vi "UHR-Fleezers Control (host) - 10.6.vi"() -> ()   [LabVIEW 2011] (continued)
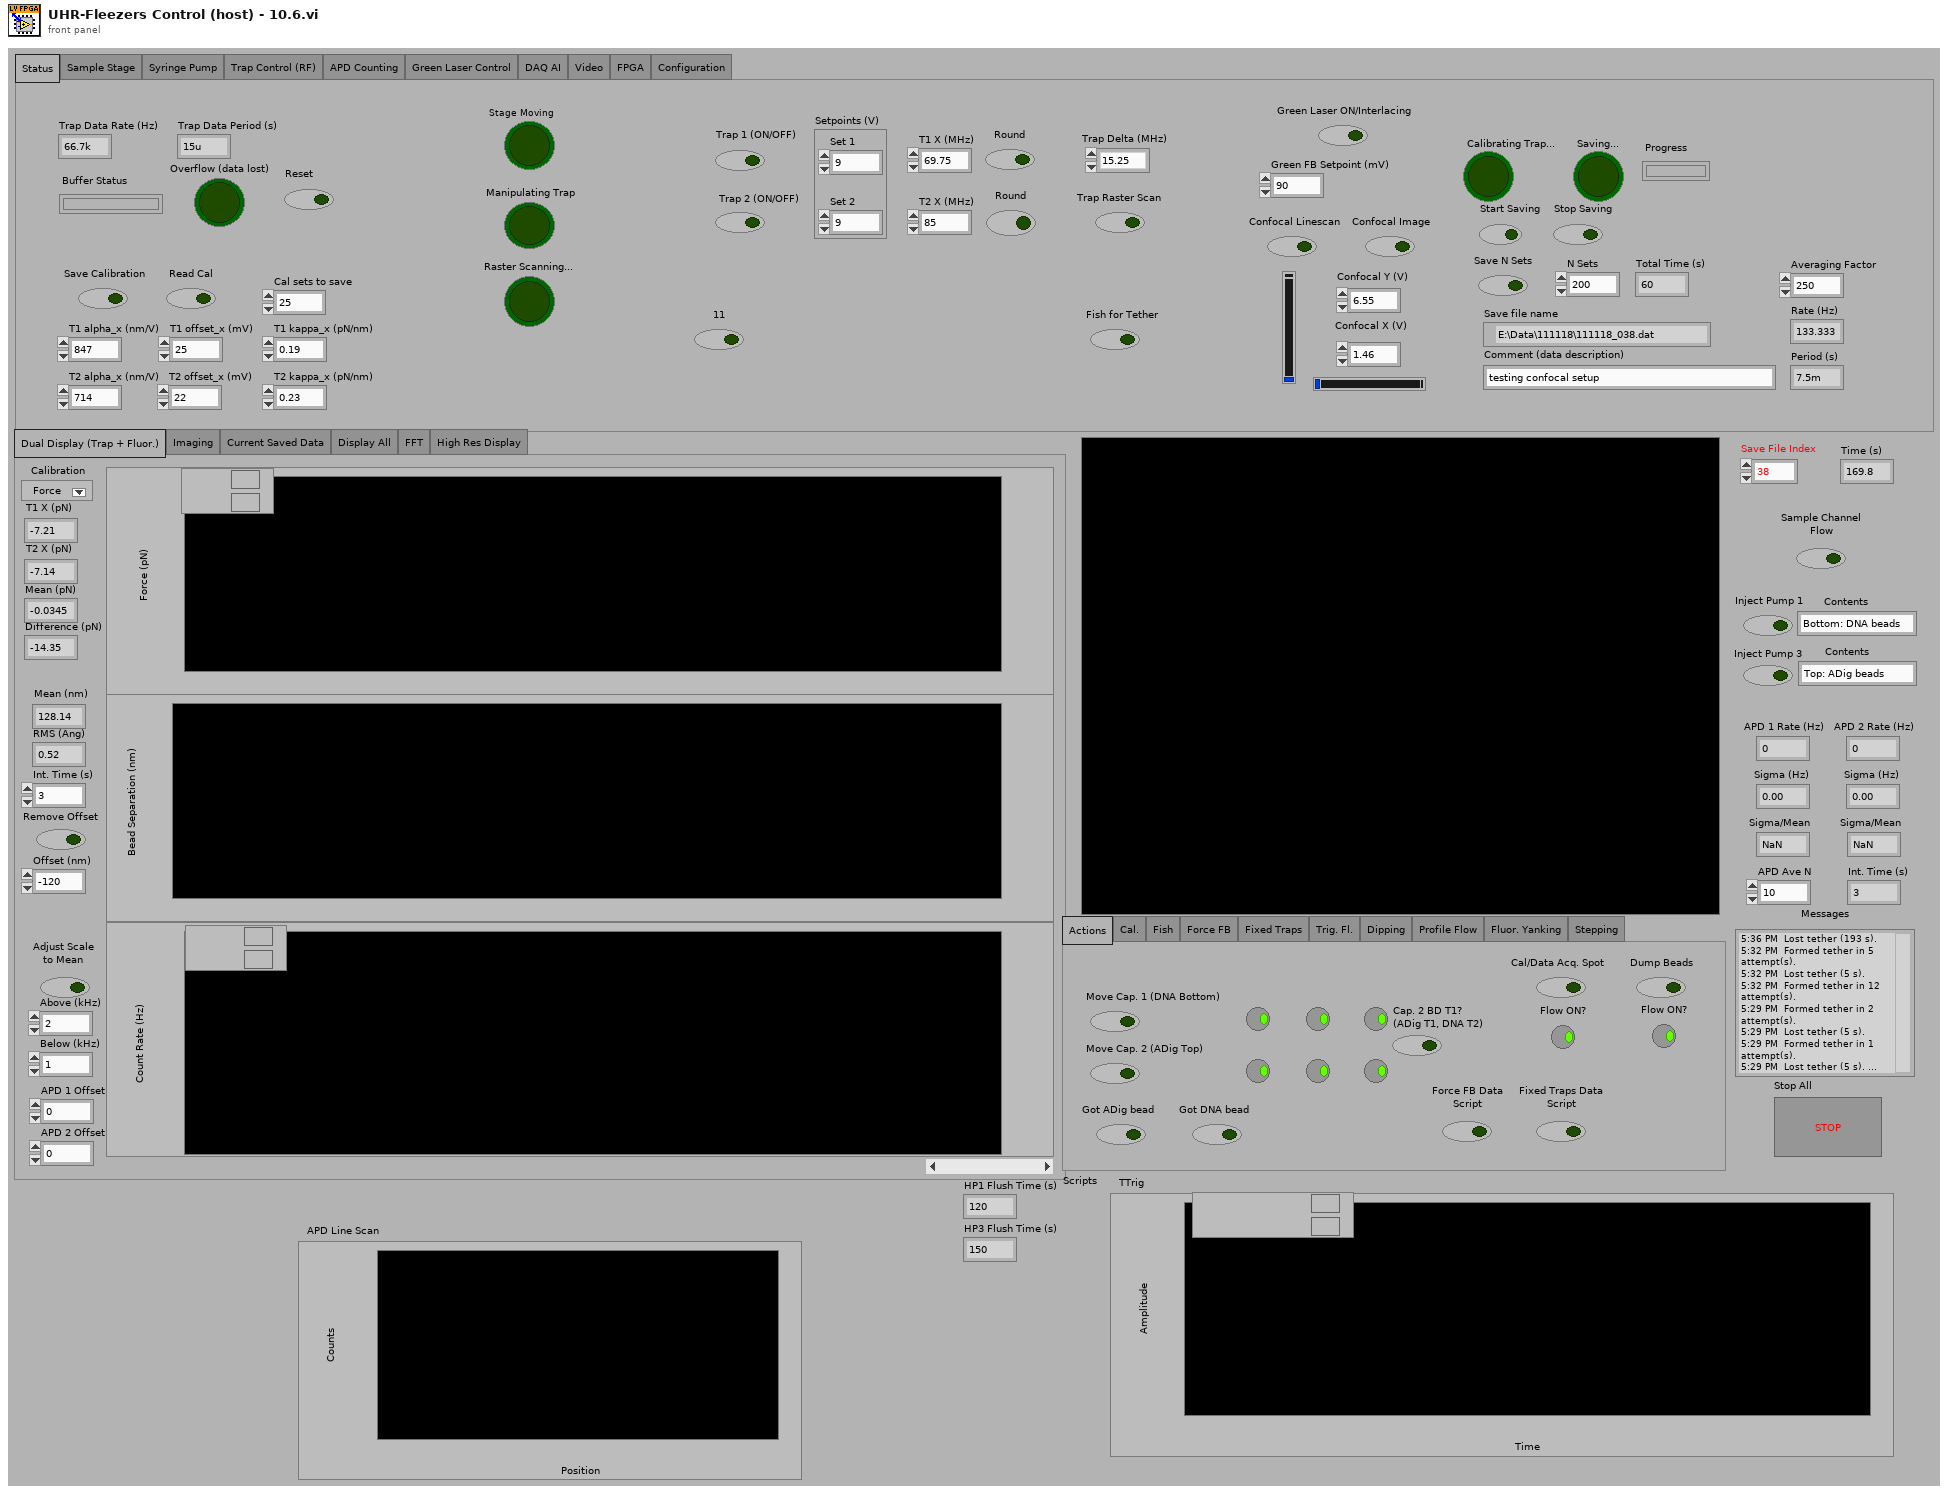
[diagram p1: front panel]
types:
  T1 = enum32{"Actions", "Cal.", "Fish", "Force FB", "Fixed Traps", "Trig. Fl.", "Dipping", "Profile Flow", "Fluor. Yanking", "Stepping"}
  T2 = typedef "IMAQ Image.ctl" = refnum<image>
  T3 = enum32{"Dual Display (Trap + Fluor.)", "Imaging", "Current Saved Data", "Display All", "FFT", "High Res Display"}
  T4 = enum32{"Status", "Sample Stage", "Syringe Pump", "Trap Control (RF)", "APD Counting", "Green Laser Control", "DAQ AI", "Video", "FPGA", "Configuration"}
  T5 = cluster{"Pump 1":cluster{"Diameter (mm)":dbl, "Units":dbl, "Volume":dbl, "Rate":dbl}, "Pump 2":cluster{"Diameter (mm)":dbl, "Units":dbl, "Volume":dbl, "Rate":dbl}, "Pump 3":cluster{"Diameter (mm)":dbl, "Units":dbl, "Volume":dbl, "Rate":dbl}}
  T6 = enum32{"IR Laser Interlacing (Direct RF Board Control Method)", "AOD Raster Scan", "Feedback on Trap Intensity", "Feedback on Trap Position"}
  T7 = typedef "LVPoint32TypeDef.ctl" = cluster{"Horizontal":i32, "Vertical":i32}
  T8 = cluster{"Scan Range AOD (nm) 2":dbl, "Step Size AOD (nm) 2":dbl, "Scan Speed AOD (nm/s) 2":dbl, "Number of scans (AOD) 2":u16, "Label":string}[]
  T9 = cluster{"Set 1":cluster{"proportional gain (Kc)":i16, "integral gain (Kc*Ts/Ti)":i16, "derivative gain (Kc*Td/Ts)":i16}, "Set 2":cluster{"proportional gain (Kc)":i16, "integral gain (Kc*Ts/Ti)":i16, "derivative gain (Kc*Td/Ts)":i16}}
  T10 = cluster{"Trap 1":fxp<+/-,16,1>, "Trap 2":fxp<+/-,16,1>}
  T11 = cluster{"proportional gain (Kc)":fxp<+/-,16,8>, "integral gain (Kc*Ts/Ti)":fxp<+/-,16,8>, "derivative gain (Kc*Td/Ts)":fxp<+/-,16,8>}
  T12 = cluster{"output high":fxp<+/-,16,1>, "output low":fxp<+/-,16,1>}
  T13 = cluster{"Set 1":fxp<+/-,16,1>, "Set 2":fxp<+/-,16,1>}
  T14 = cluster{"proportional gain (Kc)":i16, "integral gain (Kc*Ts/Ti)":i16, "derivative gain (Kc*Td/Ts)":i16}
  T15 = cluster{"Set 1":bool, "Set 2":bool, "Set 3":bool}
  T16 = typedef "LVMinMaxIncTypeDef.ctl" = cluster{"Minimum":dbl, "Maximum":dbl, "Increment":dbl}
  T17 = typedef "Image Type" = u32
  T18 = typedef "nirio_resource_hc.ctl" = tag
  T19 = typedef "openfpgaref.8.6.ctl" = refnum<k20>
  T20 = cluster{"New Image":T2, "New Image":T2, "New Image":T2, "New Image":T2}
  T21 = typedef "XDNodeRunTimeDep.lvlib/timing_clust.ctl" = cluster{"Expected End [f-1]":u64, "Actual End [f-1]":u64, "Finished Late? [f-1]":bool, "Expected End [i-1]":u64, "Actual End [i-1]":u64, "Finished Late? [i-1]":bool, "Expected Start [i]":u64, "Actual Start [i]":u64, "Expected Start [f]":u64, "Actual Start [f]":u64, "Source Name":string, "Structure Name":string, "Period":i64, "Deadline":i64, "Offset":i64, "Start":i64, "Priority":i32, "Timeout":i32, "Mode":T22, "Wakeup Reason":T23, "Error":errorcluster, "Source Type":string, "Secondary Source Type":string, "Global End Time":u64, "Global Start Time":u64, "Frame Duration":u64, "Iteration Duration":u64, "Assigned CPU":i32, "I/O Scan Engine Mode":u32}
  T22 = typedef "XDNodeRunTimeDep.lvlib/nitl_modes.ctl" = enum32{"No Change", "Process missed periods, maintain original phase", "Discard missed periods, maintain original phase", "Process missed periods, ignore original phase", "Discard missed periods, ignore original phase"}
  T23 = typedef "XDNodeRunTimeDep.lvlib/wakeup.ctl" = enum32{"Normal", "Aborted", "Asynchronous wakeup", "Timing source error", "Timed loop error", "Timeout"}
  T24 = enum16{"big-endian, network order", "native, host order", "little-endian"}
  T25 = enum16{"open", "replace", "create", "open or create", "replace or create", "replace or create with confirmation"}
  T26 = cluster{"Scan Range AOD (nm) 2":dbl, "Step Size AOD (nm) 2":dbl, "Scan Speed AOD (nm/s) 2":dbl, "Number of scans (AOD) 2":u16, "Label":string}
  T27 = cluster{"[0]":dbl, "[1]":dbl, "[2]":dbl, "[3]":dbl, "[4]":dbl, "[5]":dbl}
  T28 = cluster{"Diameter (mm)":dbl, "Units":dbl, "Volume":dbl, "Rate":dbl}
  T29 = cluster{"Left":i32, "Top":i32, "Width":u32, "Height":u32}
  T30 = cluster{cluster{"Left":i32, "Top":i32, "Width":u32, "Height":u32}}[]
  T31 = enum32{"setting", "request", "request control", "info", "statistics", "system settings", "I/O sub system", "HRT control", "camera descriptions", "device specific data", "event sub system settings", "event sub system results", "image memory manager"}
  T32 = typedef "AviRefnum.ctl" = refnum<k1>
  T33 = typedef "imagedata.ctl" = cluster{"image type":i32, "image depth":i32, "image":u8[], "mask":u8[], "colors":u32[], "Rectangle":cluster{"left":i16, "top":i16, "right":i16, "bottom":i16}}
  T34 = enum32{"Normal Display", "Dual Display (APD)", "FFT", "High Res Display"}
  T35 = cluster{"Origin Pixel":cluster{"X":sgl, "Y":sgl}, "Angle Relative to Horizontal (deg)":sgl, "Axis Reference":u32}
  T36 = typedef "Simple Grid Descriptor" = cluster{"X Step":sgl, "Y Step":sgl, "Unit":T37}
  T37 = typedef "Image Unit" = enum32{"Undefined", "Angström", "Micrometer", "Millimeter", "Centimeter", "Meter", "Kilometer", "Microinch", "Inch", "Feet", "Nautical miles", "Standard miles", "Steps"}
  T38 = cluster{"averaging mode":u16, "weighting mode":u16, "number of averages":u32}
  T39 = cluster{"dB On (F)":bool, "unwrap phase (F)":bool, "convert to degree (F)":bool}
  T40 = cluster{string, string, string, string, string, string, string, string}
  T41 = cluster{string, string, string, string, string, string, string, string, string, string, string, string}
  T42 = cluster{string, string, string, string, string, string, string, string, string, string, string, string, string}
  T43 = cluster{string, string, string, string, string, string, string, string, string, string, string, string, string, string}
  T44 = cluster{"BD 1 Frequency 1 (MHz)":dbl, "BD 1 Frequency 2 (MHz)":dbl}
  T45 = cluster{"f0":dbl, "df":dbl, "magnitude":dbl[]}[][]
  T46 = cluster{"Green FB Ch 0":i16, "Green FB Ch 1":i16, "Green FB Ch 2":i16}
  T47 = cluster{"Green FB Ch 0":dbl, "Green FB Ch 1":dbl, "Green FB Ch 2":dbl}
diagram:
  w6 = u16 20 items=["1.0"=10, "1.5"=15, "2.0"=20] ("stop bits (10: 1 bit)")
  w9 = u16 20 items=["1.0"=10, "1.5"=15, "2.0"=20] ("stop bits (10: 1 bit)")
  w67 = u16 20 items=["1.0"=10, "1.5"=15, "2.0"=20] ("stop bits (10: 1 bit)")
  w74 = T17 2 items=["Grayscale (U8)", "Grayscale (I16)", "Grayscale (SGL)", "Complex (CSG)", "RGB (U32)", "HSL (U32)", "RGB (U64)", "Grayscale (U16)"] ("Image Type")
  w137 = cluster{"output high":i16, "output low":i16} {"output high"=3000, "output low"=0} ("FB output range 1")
  w208 = 10.0 ("y")
  w207 = 32767.0 ("y")
  w223 = 6.0  # clock mult.
  w224 = 49152000.0  # TCXO frequ.
  # "Bottom 1 Harvard"
  # "Top 3 Harvard"
  # "Center Harvard"
  # "Bottom 1 Harvard"
  # "Top 3 Harvard"
  # "Center Harvard"
  n1 = Build Array("DIO count 1 (ticks)", "DIO count 2 (ticks)", "DIO count 3 (ticks)") -> (w124:u32[])
  n2 = local read "AO1"() -> (w202:dbl)
  n3 = local read "AO2"() -> (w201:dbl)
  n4 = local read "Scan Increment (MHz)"() -> (w219:dbl)
  n5 = local read "Continuous MCL Scanning"() -> (w189:bool)
  n6 = local read "Fast Scan Dir"() -> (w188:bool)
  n7 = local read "Number of scans (MCL)"() -> (w190:u64)
  n8 = property on="AI Count (ticks)" class="DigNum (strict)"("Val(Sgnl)"="AI Count (ticks)") -> ()  [unwired: 2 in, 2 out]
  n9 = Multiply(x=w202, y=w207) -> (x*y=w204:dbl)
  n10 = Multiply(x=w201, y=w207) -> (x*y=w206:dbl)
  n11 = Divide(x=w204, y=w208) -> (x/y=w203:dbl)
  n12 = Divide(x=w206, y=w208) -> (x/y=w205:dbl)
  n13 = To Word Integer(number=w203) -> (16bit integer=w200:i16)
  n14 = To Word Integer(number=w205) -> (16bit integer=w199:i16)
  n15 = Not(x=w188) -> (.not. x?=w183:bool)
  n16 = local read "Cycles/step (MCL)"() -> (w191:u64)
  n17 = Multiply(x=w219, y=1000.0) -> (x*y=w226:dbl)
  n18 = local read "Scan steps (MCL)"() -> (w192:u64)
  n19 = local write "Trap Pos FIFO Timeout"(u16 0 ("Trap Pos FIFO Timeout")) -> ()
  n20 = local read "Desired Scan Incr (V)"() -> (w194:dbl)
  n21 = Scale By Power Of 2(n=48, x=w226) -> (x*2^n=w227:dbl)
  n22 = Multiply(x=w224, y=w223) -> (x*y=w222:dbl)
  n23 = Divide(x=w227, y=w222) -> (x/y=w221:dbl)
  n24 = local read "Setpoints (V)"() -> (w240:cluster{"Set 1":dbl, "Set 2":dbl})
  n25 = To Quad Integer(1:w221) -> (0:w218:i64)
  n26 = Divide(x=40000000.0, y="AI Count (ticks)") -> (x/y=w179:dbl)
  n27 = Multiply(x=w194, y=32767.0) -> (x*y=w196:dbl)
  n28 = local read "Number Interlace Sets"() -> (w117:u8)
  n29 = Split 1D Array(array=w124, index=w117) -> (first subarray=w126:u32[])  [unwired: 1 out]
  n30 = Add Array Elements(numeric array=w126) -> (sum=w125:u32)
  n31 = local read "# Samples/channel"() -> (w211:u32)
  n32 = local read "Number of F/B Scans (AOD)"() -> (w212:u16)
  n33 = local read "Not-Interlacing Set"() -> (w116:enum32{"Set 1", "Set 2", "Set 3"})
  n34 = To Unsigned Byte Integer(number=w116) -> (unsigned 8bit integer=w122:u8)
  n35 = Index Array(array=w124, index=w122) -> (element=w123:u32)
  n36 = local read "Feedback On/Off"() -> (w243:cluster{"Set 1":bool, "Set 2":bool})
  n37 = local read "PID Gains"() -> (w235:T9)
  n38 = local read "Scan steps (AOD)"() -> (w217:u64)
  n39 = local read "All FB On/Off"() -> (w244:bool)
  n40 = local read "Cycles/step (AOD)"() -> (w216:u64)
  n41 = local write "AI rate (Hz)"(w179) -> ()
  n42 = Divide(x=w196, y=10.0) -> (x/y=w195:dbl)
  n43 = Multiply(x=w217, y=w216) -> (x*y=w215:u64)
  n44 = Multiply(x=3276.7, y=w240) -> (x*y=w239:cluster{"Set 1":dbl, "Set 2":dbl})
  n45 = xnode "FPGA Open VI Reference"("resource name"=T18 "750kHzDAQ") -> ("FPGA VI Reference Out"=w232:T19, "error out"=w231:errorcluster)  [unwired: 1 in]
  n46 = To Word Integer(number=w195) -> (16bit integer=w193:i16)
  n47 = Multiply(x=w215, y=u64 2) -> (x*y=w213:u64)
  n48 = local read "Sets to FIFO (Traps)"() -> (w247:T15)
  n49 = Divide(x=w179, y="FPGA Ave.") -> (x/y=w180:dbl)
  n50 = To Word Integer(number=w239) -> (16bit integer=w238:cluster{"Set 1":i16, "Set 2":i16})
  n51 = Unbundle By Name(w235) -> ("Set 1"=w234:T14, "Set 2"=w233:T14)
  n52 = Multiply(x=w213, y=w212) -> (x*y=w210:u64)
  n53 = local write "Ave. Rate (Hz)"(w180) -> ()
  n54 = Divide(x=w210, y=w211) -> (x/y=w209:dbl)
  n55 = Unbundle By Name(w238) -> ("Set 1"=w237:i16, "Set 2"=w236:i16)
  n56 = local read "2D or 1D Scan"() -> (w138:bool)
  n57 = local write "Data points/scans"(w210) -> ()
  n58 = local read "Scan BD"() -> (w228:bool)
  n59 = And(x=w243, y=w244) -> (x .and. y?=w242:cluster{"Set 1":bool, "Set 2":bool})
  n60 = local write "Data points/scan (f/b)"(w213) -> ()
  n61 = Reciprocal(x=w180) -> (1/x=w181:dbl)
  n62 = local read "N Acq Sets (Traps + Fl.)"() -> (w172:i16)
  n63 = local write "N sets should be saved"(w209) -> ()
  n64 = xnode "Invoke Method"("FPGA VI Reference In"=w232, "error in"=w231) -> ("FPGA VI Reference Out"=w136:T19, "error out"=w146:errorcluster)
  n65 = Unbundle By Name(w242) -> ("Set 1"=w246:bool, "Set 2"=w245:bool)
  n66 = local read "Interlace"() -> (w118:bool)
  n67 = Select(t=w125, s=w118, f=w123) -> (s? t:f=w115:u32)
  n68 = local write "Update Count (MCL)"(w115) -> ()
  n69 = local write "Total Counts (ticks)"(w115) -> ()
  n70 = local write "Ave. Period (s)"(w181) -> ()
  n71 = property on="2D or 1D Scan" class="Bool (strict)"("Val(Sgnl)"=w138) -> ()  [unwired: 2 in, 2 out]
  n72 = local read "GI Frequency, OFF count"() -> (w38:u32)
  n73 = local read "GI Frequency, ON count"() -> (w29:u32)
  n74 = local read "APD Gate OFF Count"() -> (w35:u32)
  n75 = local read "APD Gate ON Count"() -> (w31:u32)
  n76 = xnode "Read/Write Control"("FPGA VI Reference In"=w135, "error in"=w146, "ai count"="AI Count (ticks)", "Interlace ON/OFF"=w118, "Number Interlace Cycles"=w117, "AI1 Sets to FIFO"=w247, "FB On/Off Set 1"=w246, "FB On/Off Set 2"=w245, "Interlace Off Parameters"=w116, "FB Setpoint Set 1"=w237, "FB Setpoint Set 2"=w236, "FB Gains Set 1"=w234, "FB Gains Set 2"=w233, "FB output range 1"=w137, "FB output range 2"=w137, "Cycles per step"=w216, "Scan BD"=w228, "Number of scans"=w212, "Scan steps"=w217, "Scan freq.  increment"=w218, "AO1"=w200, "AO2"=w199, "Scan freq.  increment (MCL)"=w193, "Scan steps (MCL)"=w192, "Cycles per step (MCL)"=w191, "Number of scans (MCL)"=w190, "MCL count"=w115, "Cont. Scan (MCL)"=w189, "MCL Scan Axis"=w183, "1D or 2D Scan?"=w138, "N of AI1 Int Acq Sets"=w172, "Freq or Amp switch first"="Freq or Amp switch first", "Freq switch delay"="Freq switch delay", "Amp switch delay"="Amp switch delay", "Swap F1 and F2"="Swap F1 and F2", "APD to FIFO"=FALSE, "DIO count 1 (ticks)"="DIO count 1 (ticks)", "DIO count 2 (ticks)"="DIO count 2 (ticks)", "DIO count 3 (ticks)"="DIO count 3 (ticks)") -> ("FPGA VI Reference Out"=w42:T19, "error out"=w40:errorcluster)  [unwired: 1 in]
  n77 = local read "On one out of X cycles"() -> (w37:u32)
  n78 = local read "APD Integration Time (s)"() -> (w21:dbl)
  n79 = local read "DMA Update Period (s)"() -> (w20:dbl)
  n80 = Add(x=w31, y=w35) -> (x+y=w33:u32)
  n81 = Add(x=w29, y=w38) -> (x+y=w36:u32)
  n82 = local read "Green Laser ON/Interlacing"() -> (w113:bool)
  n83 = local read "Green laser mode"() -> (w114:enum32{"Laser ON", "Laser OFF", "Interlace"})
  n84 = Multiply(x=w33, y=w37) -> (x*y=w34:u32)
  n85 = Multiply(x=w37, y=w36) -> (x*y=w28:u32)
  n86 = Reciprocal(x=w21) -> (1/x=w18:dbl)
  n87 = Multiply(x=w21, y=40000000.0) -> (x*y=w17:dbl)
  n88 = Divide(x=w20, y=w21) -> (x/y=w23:dbl)
  n89 = Multiply(x="Current When FB OFF (%)", y=655.35) -> (x*y=w101:dbl)
  n90 = local read "Invert APD Gate"() -> (w27:bool)
  n91 = Multiply(x="Green FB Setpoint (mV)", y=3.2767) -> (x*y=w98:dbl)
  n92 = local read "APD Gate"() -> (w26:enum32{"ON", "OFF", "Interlace"})
  n93 = Subtract(x=w34, y=w31) -> (x-y=w32:u32)
  n94 = local write "Green FB Count"(w28) -> ()
  n95 = local write "APD Acq Rate (Hz)"(w18) -> ()
  n96 = To Unsigned Long Integer(number=w17) -> (unsigned 32bit integer=w15:u32)
  n97 = Multiply(x=2.0, y=w23) -> (x*y=w22:dbl)
  n98 = local read "Invert GI"() -> (w110:bool)
  n99 = To Unsigned Word Integer(number=w101) -> (unsigned 16bit integer=w99:u16)
  n100 = Subtract(x=w28, y=w29) -> (x-y=w30:u32)
  n101 = local write "APD Samples/FIFO Acq."(w23) -> ()
  n102 = To Word Integer(number=w98) -> (16bit integer=w96:i16)
  n103 = local write "APD Elements/DMA read"(w22) -> ()
  n104 = case shown="False" w113 {
    tunnel: w114 -> [_ w273]
    tunnel: [enum32{"Laser ON", "Laser OFF", "Interlace"}."Laser OFF" ("Green laser mode") w273] -> w109
    frame False {
    }
    frame True {
    }
  }
  n105 = local write "APD Int. Count"(w15) -> ()
  n106 = local read "Trap Pos. AI1 X Pre-scale"() -> (w53:u16)
  n107 = local read "Trap Pos FB Monitor\nT1 or T2"() -> (w60:bool)
  n108 = local read "Trap Pos FB Int Count"() -> (w46:u16)
  n109 = local read "APD 1 AO Mult."() -> (w25:i16)
  n110 = local read "Trap Pos FB Negate Action"() -> (w59:bool)
  n111 = local read "APD 2 AO Mult."() -> (w24:i16)
  n112 = local read "Trap Pos. FB Offset Factor"() -> (w58:i64)
  n113 = local read "Trap Pos. FB Mult Factor"() -> (w57:i64)
  n114 = local read "Differential FB?"() -> (w12:bool)
  n115 = local read "Neg. TTrig FPGA"() -> (w14:bool)
  n116 = local read "Trap Pos. FB Gains"() -> (w55:T11)
  n117 = local read "Trap Pos. FB Range"() -> (w56:T12)
  n118 = xnode "Read/Write Control"("FPGA VI Reference In"=w42, "error in"=w40, "Invert APD Gate"=w27, "APD Gate ON Count"=w31, "APD Gate OFF Count"=w32, "APD Acq Rate Count"=w15, "APD Gate Operating Mode"=w26, "APD 1 AO scale factor"=w25, "APD 2 AO scale factor"=w24, "Green interlace ON count"=w29, "Green interlace OFF count"=w30, "Green interlace ON count 2"=w29, "Green interlace OFF count 2"=w30, "Green FB Count"=w28) -> ("FPGA VI Reference Out"=w41:T19, "error out"=w39:errorcluster)
  n119 = xnode "Read/Write Control"("FPGA VI Reference In"=w41, "error in"=w39, "Invert GI 2"=w110, "Operating Mode 2"=w109, "Green FB Gains"="Green FB Gains", "Green FB Setpoint"=w96, "Green FB On/Off"="Green FB On/Off", "Current Out"=w99, "Green int current ON count adj"="Green int current ON count adj", "Operating Mode"=w109, "Invert GI"=w110, "Trap Pos FB Monitor T1 or T2"=w60, "Trap Pos FB Negate Action"=w59, "Trap Pos. FB Offset Factor"=w58, "Trap Pos. FB Mult Factor"=w57, "Trap Pos. FB Range"=w56, "Trap Pos. FB Gains"=w55, "Force feedback"=FALSE, "AI1 X Scale"=w53, "Trap Pos to FIFO"=TRUE, "Trap Pos FB Int Count"=w46, "TTrig Negate Pos"=w14, "FB Trig Integrate"="FB Trig Integrate", "Diff FB Measurement?"=w12, "Negate Diff?"="Negate Diff?") -> ("FPGA VI Reference Out"=w111:T19, "error out"=w112:errorcluster)
  n120 = xnode "Invoke Method"("FPGA VI Reference In"=w111, "error in"=w112, "Depth"="Trap AI FIFO Depth") -> ("FPGA VI Reference Out"=w63:T19, "error out"=w62:errorcluster)
  n121 = xnode "Invoke Method"("FPGA VI Reference In"=w63, "error in"=w62, "Depth"="Trap Position FIFO Depth") -> ("FPGA VI Reference Out"=w48:T19, "error out"=w47:errorcluster)
  n122 = flat-sequence {
    tunnel: w136 -> [w278]
    tunnel: [w278] -> w135
    tunnel: [w277] -> w134
    tunnel: [w276] -> w133
    tunnel: [w274] -> w131
    tunnel: [w275] -> w132
    frame #0 {
      w275 = T16 {"Minimum"=0.0, "Maximum"=40.0, "Increment"=1.0} ("Min Max Inc")
      w274 = T16 {"Minimum"=0.0, "Maximum"=50.0, "Increment"=1.0} ("Data Entry Limits")
      w277 = T16 {"Minimum"=60.0, "Maximum"=90.0, "Increment"=1.0} ("Min Max Inc")
      w276 = T16 {"Minimum"=0.0, "Maximum"=50.0, "Increment"=1.0} ("Data Entry Limits")
      n123 = property on="BD 2 Frequency 1 (MHz)" class="DigNum (strict)"("Data Range"=w275) -> ()  [unwired: 2 in, 2 out]
      n124 = property on="BD 2 Frequency 3 (MHz)" class="DigNum (strict)"("Data Range"=w275) -> ()  [unwired: 2 in, 2 out]
      n125 = property on="BD 2 Frequency 2 (MHz)" class="DigNum (strict)"("Data Range"=w275) -> ()  [unwired: 2 in, 2 out]
      n126 = property on="BD 1 Frequency 1 (MHz)" class="DigNum (strict)"("Data Range"=w277) -> ()  [unwired: 2 in, 2 out]
      n127 = property on="BD 1 Frequency 2 (MHz)" class="DigNum (strict)"("Data Range"=w277) -> ()  [unwired: 2 in, 2 out]
      n128 = property on="BD 1 Frequency 3 (MHz)" class="DigNum (strict)"("Data Range"=w277) -> ()  [unwired: 2 in, 2 out]
      n129 = property on="BD 2 Amplitude 1 (%)" class="DigNum (strict)"("Data Range"=w274) -> ()  [unwired: 2 in, 2 out]
      n130 = property on="BD 2 Amplitude 2 (%)" class="DigNum (strict)"("Data Range"=w274) -> ()  [unwired: 2 in, 2 out]
      n131 = property on="BD 2 Amplitude 3 (%)" class="DigNum (strict)"("Data Range"=w274) -> ()  [unwired: 2 in, 2 out]
      n132 = property on="BD 1 Amplitude 3 (%)" class="DigNum (strict)"("Data Range"=w276) -> ()  [unwired: 2 in, 2 out]
      n133 = property on="BD 1 Amplitude 2 (%)" class="DigNum (strict)"("Data Range"=w276) -> ()  [unwired: 2 in, 2 out]
      n134 = property on="BD 1 Amplitude 1 (%)" class="DigNum (strict)"("Data Range"=w276) -> ()  [unwired: 2 in, 2 out]
      "X RF Frequency Limits (MHz)" <- w277
      "X RF Amplitude Limits (%)" <- w276
      "Y RF Amplitude Limits (%)" <- w274
      "Y RF Frequency Limits (MHz)" <- w275
    }
  }
  n135 = xnode "Invoke Method"("FPGA VI Reference In"=w48, "error in"=w47) -> ("FPGA VI Reference Out"=w145:T19, "error out"=w144:errorcluster)  [unwired: 1 in]
  n136 = flat-sequence "Initial FPGA Loop Relative Phase Adjustment" {
    tunnel: "Initial Phase Adjustment (AI1)" -> [w289]
    tunnel: "Initial Phase Adjustment (GI)" -> [w288]
    tunnel: w145 -> [w287]
    tunnel: w144 -> [w286]
    tunnel: "Initial Phase Adj. (MCL)" -> [w285]
    tunnel: [w290] -> w154
    tunnel: [w284] -> w150
    tunnel: "Initial Phase Adjustment (APD Acq)" -> [w283]
    tunnel: "Initial Phase Adjustment (APD 1 Gate)" -> [w282]
    tunnel: "Initial Phase Adjustment (Green FB)" -> [w281]
    tunnel: "Initial Phase Adjustment (GI) 2" -> [w280]
    tunnel: "Initial Phase Adjustment (APD 2 Gate)" -> [w279]
    tunnel: w154 -> [w292]
    tunnel: [w293] -> w151
    tunnel: w150 -> [w293]
    tunnel: [w292] -> w149
    tunnel: w151 -> [w296]
    tunnel: w149 -> [w295]
    tunnel: [w298] -> w148
    tunnel: [w297] -> w147
    tunnel: [w300] -> w152
    tunnel: [w301] -> w153
    tunnel: w148 -> [w301]
    tunnel: w147 -> [w300]
    frame #0 {
      n137 = xnode "Read/Write Control"("FPGA VI Reference In"=w287, "error in"=w286, "Phase count adjustment"=w289, "Phase count adjustment (GI)"=w288, "Phase count adjustment (MCL)"=w285, "Phase Count Adjustment (APD Acq)"=w283, "Phase count adjustment (APD 1 Gate)"=w282, "Phase count adjustment (APD 2 Gate)"=w279, "Phase count adjustment (Green FB)"=w281, "Phase count adjustment (GI) 2"=w280) -> ("FPGA VI Reference Out"=w284:T19, "error out"=w290:errorcluster)
    }
    frame #1 {
      n138 = Wait (ms)(milliseconds to wait=u32 100) -> ()  [unwired: 1 out]
    }
    frame #2 {
      w294 = TRUE
      n139 = xnode "Read/Write Control"("FPGA VI Reference In"=w296, "error in"=w295, "+ phase"=w294, "+ phase (GI)"=w294, "+ phase (MCL)"=w294, "+ phase (APD Acq)"=w294, "+ phase (APD 1 Gate)"=w294, "+ phase (APD 2 Gate)"=w294, "+ phase (Green FB)"=w294, "+ phase (GI) 2"=w294) -> ("FPGA VI Reference Out"=w297:T19, "error out"=w298:errorcluster)
    }
    frame #3 {
      n140 = Wait (ms)(milliseconds to wait=u32 100) -> ()  [unwired: 1 out]
    }
  }
  n141 = local read "Phase adj. (Green FB)"() -> (w127:i16)
  n142 = local read "Phase adj. (GI) 2"() -> (w102:i16)
  n143 = local read "Phase adjust (MCL)"() -> (w184:i16)
  n144 = local read "Phase adj. (AI1)"() -> (w186:i16)
  n145 = local read "Phase adj. (GI)"() -> (w185:i16)
  n146 = xnode "Read/Write Control"("FPGA VI Reference In"=w152, "error in"=w153, "Phase count adjustment"=w186, "Phase count adjustment (GI)"=w185, "Phase count adjustment (MCL)"=w184, "Phase Count Adjustment (APD Acq)"="Phase Adj. (APD Acq)", "Phase count adjustment (APD 1 Gate)"="Phase Adj. (APD 1 Gate)", "Phase count adjustment (APD 2 Gate)"="Phase Adj. (APD 2 Gate)", "Phase count adjustment (Green FB)"=w127, "Phase count adjustment (GI) 2"=w102) -> ("FPGA VI Reference Out"=w88:T19, "error out"=w161:errorcluster)
  n147 = call "Initialize RF boards - interlace 3.vi"("error in"=w161, "FPGA VI Reference In"=w88) -> ("error out"=w159:errorcluster, "FPGA VI Reference Out"=w160:T19)
  n148 = call "set RF board frequency - interlace.vi"("Board 2 Frequency Limits"=w132, "Board 1 Frequency Limits"=w134, "error in"=w159, "FPGA VI Reference In"=w160, "Board 2 Frequency 3 (MHz)"="BD 2 Frequency 3 (MHz)", "Board 1 Frequency 3 (MHz)"="BD 1 Frequency 3 (MHz)", "Board 2 Frequency 2 (MHz)"="BD 2 Frequency 2 (MHz)", "Board 2 Frequency 1 (MHz)"="BD 2 Frequency 1 (MHz)", "Board 1 Frequency 2 (MHz)"="BD 1 Frequency 2 (MHz)", "Board 1 Frequency 1  (MHz)"="BD 1 Frequency 1 (MHz)") -> ("error out"=w262:errorcluster, "FPGA VI Reference Out"=w263:T19)
  n149 = call "set RF board amplitude - interlace.vi"("Board 2 Amplitude Limits"=w131, "Board 1 Amplitude Limits"=w133, "error in"=w262, "FPGA VI Reference In"=w263, "Board 2 Amplitude 3 (%)"="BD 2 Amplitude 3 (%)", "Board 1 Amplitude 3 (%)"="BD 1 Amplitude 3 (%)", "Board 2 Amplitude 2 (%)"="BD 2 Amplitude 2 (%)", "Board 2 Amplitude 1 (%)"="BD 2 Amplitude 1 (%)", "Board 1 Amplitude 2 (%)"="BD 1 Amplitude 2 (%)", "Board 1 Amplitude 1 (%)"="BD 1 Amplitude 1 (%)") -> ("error out"=w250:errorcluster, "FPGA VI Reference Out"=w251:T19)
  n150 = flat-sequence {
    tunnel: w251 -> [w311]
    tunnel: w250 -> [w310]
    tunnel: [w309] -> w255
    tunnel: [w308] -> w254
    tunnel: [w315] -> w253
    tunnel: w255 -> [w315]
    tunnel: [w314] -> w252
    tunnel: w254 -> [w314]
    tunnel: w253 -> [w324]
    tunnel: w252 -> [w323]
    tunnel: [w322] -> w50
    tunnel: [w321] -> w49
    frame #0 {
      w302 = FALSE ("Retract Pump 3")
      n151 = local read "Trap 1 (ON/OFF)"() -> (w303:bool)
      n152 = xnode "Read/Write Control"("FPGA VI Reference In"=w311, "error in"=w310, "Direct RF Box  Communication"=FALSE) -> ("FPGA VI Reference Out"=w309:T19, "error out"=w308:errorcluster)
      n153 = local write "Saving..."(FALSE ("Saving Data")) -> ()
      n154 = local write "Stop All"(FALSE ("Stop All")) -> ()
      n155 = local write "Retract Pump 1"(w302) -> ()
      n156 = local write "Retract Pump 3"(w302) -> ()
      n157 = local write "Index"(1.0 ("Index")) -> ()
      n158 = property on="Trap 1 ON" class="Bool (strict)"("Value"=w303) -> ()  [unwired: 2 in, 2 out]
      "Manipulating Trap" <- FALSE ("Manipulating Trap")
    }
    frame #1 {
      n159 = local read "Trap 2 (ON/OFF)"() -> (w313:bool)
      n160 = Wait (ms)(milliseconds to wait=u32 10) -> ()  [unwired: 1 out]
      n161 = property on="Trap 2 ON" class="Bool (strict)"("Val(Sgnl)"=w313) -> ()  [unwired: 2 in, 2 out]
    }
    frame #2 {
      n162 = local read "Scan Range (nm)"() -> (w317:dbl)
      n163 = xnode "Read/Write Control"("FPGA VI Reference In"=w324, "error in"=w323, "FPGA Controls  RF Box"=TRUE ("Direct RF Box  Communication")) -> ("FPGA VI Reference Out"=w322:T19, "error out"=w321:errorcluster)
      n164 = call "Update messages.vi"("Message to add"="UHR-Fleezers ready.", "Old message string"="") -> ("New message string"=w320:string)
      n165 = local write "Messages"(w320) -> ()
      n166 = property on="Scan Range (nm)" class="DigNum (strict)"("Val(Sgnl)"=w317) -> ()  [unwired: 2 in, 2 out]
    }
  }
  n167 = Subtract(x="BD 1 Frequency 1 (MHz)", y="BD 1 Frequency 2 (MHz)") -> (x-y=w171:dbl)
  n168 = Subtract(x="BD 2 Frequency 1 (MHz)", y="BD 2 Frequency 2 (MHz)") -> (x-y=w170:dbl)
  n169 = Square(x=w170) -> (x^2=w168:dbl)
  n170 = Square(x=w171) -> (x^2=w169:dbl)
  n171 = Add(x=w169, y=w168) -> (x+y=w167:dbl)
  n172 = Square Root(x=w167) -> (sqrt(x)=w166:dbl)
  n173 = local write "Trap Delta (MHz)"(w166) -> ()
  n174 = call "IMAQ Create"("Image Name"="APD 1 Image", "Image Type"=w74) -> ("New Image"=w73:T2)  [unwired: 3 in, 1 out]
  n175 = call "IMAQ Create"("Image Name"="APD 2 Image", "Image Type"=w74) -> ("New Image"=w72:T2)  [unwired: 3 in, 1 out]
  n176 = call "IMAQ Create"("Image Name"="Det. X Image", "Image Type"=w74) -> ("New Image"=w71:T2)  [unwired: 3 in, 1 out]
  n177 = call "IMAQ Create"("Image Name"="Det. Y Image", "Image Type"=w74) -> ("New Image"=w70:T2)  [unwired: 3 in, 1 out]
  n178 = Bundle("New Image"=w73, "New Image"=w72, "New Image"=w71, "New Image"=w70) -> (w69:T20)  [unwired: 1 in]
  n179 = call-poly "VISA Configure Serial Port"("VISA resource name"="Bottom  1 Harvard Syringe Pump Serial Port", "baud rate (9600)"=u32 115200, "stop bits (10: 1 bit)"=w6) -> ("VISA resource name out"=w2:refnum<visa-resource-name>, "error out"=w1:errorcluster)  [unwired: 4 in, 7 out]
  n180 = call-poly "VISA Configure Serial Port"("VISA resource name"="Top 3 Harvard Syringe Pump Serial Port", "baud rate (9600)"=u32 115200, "stop bits (10: 1 bit)"=w9) -> ("VISA resource name out"=w4:refnum<visa-resource-name>, "error out"=w3:errorcluster)  [unwired: 4 in, 7 out]
  n181 = call-poly "VISA Configure Serial Port"("VISA resource name"="Sample Chamber Stage Serial Port") -> ("VISA resource name out"=w83:refnum<visa-resource-name>, "error out"=w84:errorcluster)  [unwired: 5 in, 8 out]
  "Stage Control Serial Error" <- w84
  n182 = call-poly "VISA Configure Serial Port"("VISA resource name"="Center Harvard Syringe Pump Serial Port", "baud rate (9600)"=u32 115200, "stop bits (10: 1 bit)"=w67) -> ("VISA resource name out"=w64:refnum<visa-resource-name>, "error out"=w65:errorcluster)  [unwired: 4 in, 7 out]
  n183 = node-c288() -> (w79:T21)  [unwired: 4 in]
  n184 = timed-loop "Run Scripts, including: stage motion" {
    tunnel: w84 -> [w332]
    tunnel: w83 -> [w333]
    tunnel: [w333] -> w82
    tunnel: [w332] -> w81
    timing: w79 -> [_]
    timing-out: [_] -> w78
    tunnel: w64 -> [w331]
    tunnel: w65 -> [w330]
    tunnel: w4 -> [w327]
    tunnel: w3 -> [w326]
    tunnel: w2 -> [w328]
    tunnel: w1 -> [w329]
    stop <- w334 stop-if-true
    n185 = node-c288() -> ()  [unwired: 1 in, 1 out]
    n186 = event shown="[2] \"Move Cap. 1 (DNA Bottom)\": Value Change" {
      selector: _ -> [_ _ _ _ _ _ _ _ _ _ _ _ _ _ _ _ _ _ _]
      dyn-events: _ -> [_ _ _ _ _ _ _ _ _ _ _ _ _ _ _ _ _ _ _]
      timeout: _ -> [_ _ _ _ _ _ _ _ _ _ _ _ _ _ _ _ _ _ _]
      tunnel: ["Set Position" "Move to Position" _ _ "Read Harvard" _ _ _ _ _ _ "Got ADig bead" "Force FB Data\nScript" _ "Got DNA bead" "Take Stepping Data" _ "Take Detection Laser\nImage" _] -> _
      tunnel: [_ _ _ _ _ _ _ _ _ _ _ _ _ _ _ _ _ _ w951] -> w334
      tunnel: w332 -> [w352 w360 w373 w403 _ w448 w488 w569 w598 w730 w756 _ w792 _ _ _ _ _ _]
      tunnel: w333 -> [w353 w361 w374 w404 _ w449 w489 w570 w599 w731 w757 _ w793 _ _ _ _ _ _]
      tunnel: w331 -> [_ _ _ _ w433 _ _ _ _ _ _ _ _ _ _ _ _ _ _]
      tunnel: w330 -> [_ _ _ _ w432 _ _ _ _ _ _ _ _ _ _ _ _ _ _]
      tunnel: w329 -> [_ _ _ _ _ _ _ _ _ _ _ _ _ _ _ _ _ _ _]
      tunnel: w328 -> [_ _ _ _ _ _ _ _ _ _ _ _ _ _ _ _ _ _ _]
      tunnel: w327 -> [_ _ _ _ _ _ _ _ _ _ _ _ _ _ _ _ _ _ _]
      tunnel: w326 -> [_ _ _ _ _ _ _ _ _ _ _ _ _ _ _ _ _ _ _]
      event "Set Position", "Set Position 2", "Set Position 3", "Set Position 4", "Set Position 5", "Set Position 1": Value Change {
        n187 = event-data() -> ()  [unwired: 1 in, 5 out]
        n188 = Build Array("Set Position 1", "Set Position 2", "Set Position 3", "Set Position 4", "Set Position 5") -> (w351:bool[])
        n189 = Boolean Array To Number(Boolean array=w351) -> (number=w350:u32)
        n190 = Logarithm Base 2(1:w350) -> (0:w342:dbl)
        n191 = call "Read Stage Position.vi"("error in"=w352, "VISA resource name in"=w353) -> ("Current Position"=w357:cluster{dbl, dbl, dbl}, "error out"=w356:errorcluster)  [unwired: 2 out]
        n192 = Decrement(x="Position") -> (x-1=w340:dbl)
        n193 = Greater Or Equal?(x=w342, y=0.0) -> (x >= y?=w343:bool)
        n194 = Cluster To Array(cluster=w357) -> (array=w354:dbl[])
        n195 = local write "Stage Control Serial Error"(w356) -> ()
        n196 = Select(t=w342, s=w343, f=w340) -> (s? t:f=w339:dbl)
        n197 = Increment(x=w339) -> (x+1=w338:dbl)
        n198 = Build Array (concatenate)(w338, w354) -> (w337:dbl[])
        n199 = Replace Array Subset(array="Saved Stage Positions", new element=w337, index (row)=w339) -> (w355:dbl[][])  [unwired: 1 in]
        n200 = local write "Saved Stage Positions"(w355) -> ()
      }
      event "Move to Position": Value Change {
        n201 = event-data() -> ()  [unwired: 1 in, 5 out]
        n202 = flat-sequence {
          tunnel: w361 -> [w365]
          tunnel: w360 -> [w364]
          frame #0 {
            n203 = local read "Saved Stage Positions"() -> (w367:dbl[][])
            n204 = local read "Position"() -> (w366:dbl)
            n205 = local write "Stage Moving"(TRUE ("Stage Moving")) -> ()
            n206 = call "move to saved stage position.vi"("error in"=w364, "Stage VISA resource name in"=w365, "Position"=w366, "Saved Stage Positions"=w367) -> ("error out"=w363:errorcluster)  [unwired: 1 out]
            n207 = local write "Stage Control Serial Error"(w363) -> ()
          }
          frame #1 {
            n208 = call <vilib>:"Beep.vi"() -> ()  [unwired: 3 in, 9 out]
            n209 = local write "Stage Moving"(FALSE ("Stage Moving")) -> ()
          }
        }
      }
      event "Move Cap. 1 (DNA Bottom)": Value Change {
        n210 = event-data() -> ()  [unwired: 1 in, 5 out]
        n211 = local write "Move Cap. 1 (DNA Bottom)"(FALSE ("Move Cap. 1 (DNA Right)")) -> ()
        n212 = flat-sequence {
          tunnel: w373 -> [w376]
          tunnel: w374 -> [w377]
          tunnel: [w377] -> w371
          tunnel: [w376] -> w370
          tunnel: w371 -> [w379]
          tunnel: w370 -> [w378]
          frame #0 {
            n213 = property on="Sample Channel\nFlow" class="Bool (strict)"("Val(Sgnl)"="Cap 1 Samp Flow ON") -> ()  [unwired: 2 in, 2 out]
          }
          frame #1 {
            n214 = local read "Saved Stage Positions"() -> (w389:dbl[][])
            n215 = local write "Stage Moving"(TRUE ("Stage Moving")) -> ()
            n216 = Array Subset(array=w389, index (row)=0 ("index"), length (row)=1 ("length"), index (col)=1 ("index"), length (col)=3 ("length")) -> (w386:dbl[][])
            n217 = Reshape Array(w386, 3 ("dimension size")) -> (w384:dbl[])
            n218 = Array To Cluster(array=w384) -> (cluster=w383:cluster{"[0]":dbl, "[1]":dbl, "[2]":dbl})
            n219 = call "Set Stage Position.vi"("Position"=w383, "error in"=w378, "VISA resource name in"=w379) -> ("error out"=w382:errorcluster)  [unwired: 2 out]
            n220 = local write "Stage Control Serial Error"(w382) -> ()
          }
          frame #2 {
            n221 = local write "Stage Moving"(FALSE ("Stage Moving")) -> ()
            n222 = case shown="True" "Cap 1 Flow ON" {
              frame False {
              }
              frame True {
                n223 = property on="Inject Pump 1" class="Bool (strict)"("Val(Sgnl)"=TRUE ("Value (Signaling)")) -> ()  [unwired: 2 in, 2 out]
              }
            }
            n224 = call <vilib>:"Beep.vi"() -> ()  [unwired: 3 in, 9 out]
          }
          frame #3 {
            n225 = property on="Sample Channel\nFlow" class="Bool (strict)"("Val(Sgnl)"=FALSE ("Value (Signaling)")) -> ()  [unwired: 2 in, 2 out]
            n226 = local read "Cap. 2 BD T1?\n(ADig T1, DNA T2)"() -> (w396:bool)
            n227 = case shown="True" w396 {
              tunnel: "Cap 1 T ON" -> [w398 w399]
              frame False {
                n228 = property on="Trap 1 (ON/OFF)" class="Bool (strict)"("Val(Sgnl)"=w398) -> ()  [unwired: 2 in, 2 out]
              }
              frame True {
                n229 = property on="Trap 2 (ON/OFF)" class="Bool (strict)"("Val(Sgnl)"=w399) -> ()  [unwired: 2 in, 2 out]
              }
            }
            n230 = property on="Got DNA bead" class="Bool"("Key Focus"=TRUE) -> ()  [unwired: 2 in, 2 out]
          }
        }
      }
      event "Move Cap. 2 (ADig Top)": Value Change {
        n231 = event-data() -> ()  [unwired: 1 in, 5 out]
        n232 = local write "Move Cap. 2 (ADig Top)"(FALSE ("Move Cap. 2 (ADig Left)")) -> ()
        n233 = flat-sequence {
          tunnel: w403 -> [w406]
          tunnel: w404 -> [w407]
          tunnel: [w407] -> w401
          tunnel: [w406] -> w400
          tunnel: w401 -> [w410]
          tunnel: w400 -> [w409]
          frame #0 {
            n234 = property on="Sample Channel\nFlow" class="Bool (strict)"("Val(Sgnl)"="Cap 2 Samp Flow ON") -> ()  [unwired: 2 in, 2 out]
          }
          frame #1 {
            w408 = FALSE ("Value (Signaling)")
            n235 = local read "Saved Stage Positions"() -> (w420:dbl[][])
            n236 = local write "Stage Moving"(TRUE ("Stage Moving")) -> ()
            n237 = Array Subset(array=w420, index (row)=1 ("index"), length (row)=1 ("length"), index (col)=1 ("index"), length (col)=3 ("length")) -> (w417:dbl[][])
            n238 = Reshape Array(w417, 3 ("dimension size")) -> (w415:dbl[])
            n239 = property on="Trap 1 (ON/OFF)" class="Bool (strict)"("Val(Sgnl)"=w408) -> ()  [unwired: 2 in, 2 out]
            n240 = property on="Trap 1 (ON/OFF)" class="Bool (strict)"("Val(Sgnl)"=w408) -> ()  [unwired: 2 in, 2 out]
            n241 = Array To Cluster(array=w415) -> (cluster=w414:cluster{"[0]":dbl, "[1]":dbl, "[2]":dbl})
            n242 = call "Set Stage Position.vi"("Position"=w414, "error in"=w409, "VISA resource name in"=w410) -> ("error out"=w413:errorcluster)  [unwired: 2 out]
            n243 = local write "Stage Control Serial Error"(w413) -> ()
          }
          frame #2 {
            n244 = local write "Stage Moving"(FALSE ("Stage Moving")) -> ()
            n245 = call <vilib>:"Beep.vi"() -> ()  [unwired: 3 in, 9 out]
            n246 = case shown="True" "Cap 2 Flow ON" {
              frame False {
              }
              frame True {
                n247 = property on="Inject Pump 3" class="Bool (strict)"("Val(Sgnl)"=TRUE ("Value (Signaling)")) -> ()  [unwired: 2 in, 2 out]
              }
            }
          }
          frame #3 {
            n248 = property on="Sample Channel\nFlow" class="Bool (strict)"("Val(Sgnl)"=FALSE ("Value (Signaling)")) -> ()  [unwired: 2 in, 2 out]
            n249 = case shown="False" "Cap. 2 BD T1?\n(ADig T1, DNA T2)" {
              tunnel: "Cap 2 T ON" -> [w429 w430]
              frame False {
                n250 = property on="Trap 2 (ON/OFF)" class="Bool (strict)"("Val(Sgnl)"=w429) -> ()  [unwired: 2 in, 2 out]
              }
              frame True {
                n251 = property on="Trap 1 (ON/OFF)" class="Bool (strict)"("Val(Sgnl)"=w430) -> ()  [unwired: 2 in, 2 out]
              }
            }
            n252 = property on="Got ADig bead" class="Bool"("Key Focus"=TRUE) -> ()  [unwired: 2 in, 2 out]
          }
        }
      }
      event "Read Harvard": Value Change {
        n253 = event-data() -> ()  [unwired: 1 in, 5 out]
        n254 = Concatenate Strings("write buffer", "\r") -> (w435:string)
        n255 = VISA Write(VISA resource name=w433, write buffer=w435, error in (no error)=w432) -> (VISA resource name out=w444:refnum<visa-resource-name>, error out=w443:errorcluster)  [unwired: 1 out]
        n256 = stacked-sequence {
          tunnel: [w447] -> w442
          tunnel: w444 -> [w447]
          tunnel: w443 -> [w446]
          tunnel: [w446] -> w437
          frame #0 {
            n257 = Wait (ms)(milliseconds to wait=50) -> ()  [unwired: 1 out]
          }
        }
        n258 = property class="Instr"(reference=w442, error in=w437) -> (reference out=w441:refnum<visa-resource-name>, error out=w439:errorcluster, "Serial Settings:Number of Bytes at Serial Port"=w440:u32)
        "Serial Settings:Number of Bytes at Serial Port" <- w440
        n259 = VISA Read(VISA resource name=w441, byte count=w440, error in (no error)=w439) -> (read buffer=w438:string)  [unwired: 3 out]
        "read buffer" <- w438
        n260 = Fract/Exp String To Number(string=w438) -> ()  [unwired: 5 out]
      }
      event "+z", "-z": Value Change {
        n261 = event-data() -> ()  [unwired: 1 in, 5 out]
        n262 = flat-sequence {
          tunnel: w448 -> [w470]
          tunnel: w449 -> [w450]
          frame #0 {
            n263 = call "Read Stage Position.vi"("error in"=w470, "VISA resource name in"=w450) -> ("Current Position"=w455:cluster{dbl, dbl, dbl}, "error out"=w468:errorcluster, "VISA resource name out"=w469:refnum<visa-resource-name>)  [unwired: 1 out]
            n264 = local read "Saved Stage Positions"() -> (w479:dbl[][])
            n265 = Divide(x="z nudge increment (um)", y=1000.0) -> (x/y=w467:dbl)
            n266 = Boolean To (0,1)(Boolean="+z") -> (0, 1=w459:i16)
            n267 = Boolean To (0,1)(Boolean="-z") -> (0, 1=w460:i16)
            n268 = Array Subset(array=w479, index (row)=1 ("index"), length (row)=1 ("length"), index (col)=1 ("index"), length (col)=3 ("length")) -> (w476:dbl[][])
            n269 = Multiply(x=w459, y=w467) -> (x*y=w463:dbl)
            n270 = Multiply(x=w460, y=w467) -> (x*y=w461:dbl)
            n271 = Unbundle(w455) -> (w453:dbl, w452:dbl, w456:dbl)
            n272 = Negate(x=w461) -> (-x=w462:dbl)
            n273 = Reshape Array(w476, 3 ("dimension size")) -> (w474:dbl[])
            n274 = Add(x=w463, y=w462) -> (x+y=w464:dbl)
            n275 = Array To Cluster(array=w474) -> ()  [unwired: 1 out]
            n276 = Add(x=w464, y=w456) -> (x+y=w454:dbl)
            n277 = Bundle(cluster=w455, w453, w452, w454) -> (w451:cluster{dbl, dbl, dbl})
            n278 = call "Set Stage Position.vi"("Position"=w451, "error in"=w468, "VISA resource name in"=w469) -> ("error out"=w473:errorcluster)  [unwired: 2 out]
            n279 = local write "Stage Moving"(TRUE ("Stage Moving")) -> ()
            n280 = local write "Stage Control Serial Error"(w473) -> ()
          }
          frame #1 {
            n281 = local write "Stage Moving"(FALSE ("Stage Moving")) -> ()
            n282 = call <vilib>:"Beep.vi"() -> ()  [unwired: 3 in, 9 out]
          }
        }
      }
      event "Cal/Data Acq. Spot": Value Change {
        n283 = event-data() -> ()  [unwired: 1 in, 5 out]
        n284 = flat-sequence {
          tunnel: w488 -> [w492]
          tunnel: w489 -> [w493]
          tunnel: [w493] -> w485
          tunnel: [w492] -> w484
          tunnel: w485 -> [w498]
          tunnel: w484 -> [w497]
          tunnel: ["Cal @ (MHz)"] -> w482
          tunnel: [w502] -> w486
          tunnel: w482 -> [w502]
          tunnel: w486 -> [w511]
          tunnel: ["W/ Offset 1"] -> w483
          tunnel: w486 -> [w532]
          tunnel: w483 -> [w530]
          frame #0 {
            n285 = property on="Sample Channel\nFlow" class="Bool (strict)"("Val(Sgnl)"="Daq spot flow on") -> ()  [unwired: 2 in, 2 out]
            n286 = Wait (ms)(milliseconds to wait=u32 250) -> ()  [unwired: 1 out]
          }
          frame #1 {
            n287 = local read "Saved Stage Positions"() -> (w495:dbl[][])
            n288 = property on="Trap Delta (MHz)" class="DigNum (strict)"("Val(Sgnl)"="Cal @ (MHz)") -> ()  [unwired: 2 in, 2 out]
            n289 = local write "Stage Moving"(TRUE ("Stage Moving")) -> ()
            n290 = call "move to saved stage position.vi"("error in"=w497, "Stage VISA resource name in"=w498, "Position"="Cal Stage Position", "Saved Stage Positions"=w495) -> ("error out"=w496:errorcluster)  [unwired: 1 out]
            n291 = local write "Stage Control Serial Error"(w496) -> ()
          }
          frame #2 {
            n292 = local write "Stage Moving"(FALSE ("Stage Moving")) -> ()
            n293 = property on="Sample Channel\nFlow" class="Bool (strict)"("Val(Sgnl)"="Flow ON during cal?") -> ()  [unwired: 2 in, 2 out]
            n294 = call <vilib>:"Beep.vi"() -> ()  [unwired: 3 in, 9 out]
          }
          frame #3 {
            n295 = Wait (ms)(milliseconds to wait=u32 1000) -> ()  [unwired: 1 out]
          }
          frame #4 {
            n296 = property on="Save Calibration" class="Bool (strict)"("Val(Sgnl)"=TRUE ("Value (Signaling)")) -> ()  [unwired: 2 in, 2 out]
          }
          frame #5 {
            n297 = Wait (ms)(milliseconds to wait=u32 2000) -> ()  [unwired: 1 out]
          }
          frame #6 {
            # "Check to see if \nsaving done"
            n298 = while {
              stop <- w507 stop-if-true
              n299 = local read "Saving..."() -> (w508:bool)
              n300 = Wait (ms)(milliseconds to wait=u32 100) -> ()  [unwired: 1 out]
              n301 = Not(x=w508) -> (.not. x?=w507:bool)
            }
          }
          frame #7 {
            n302 = case shown="True" "W/ Offset 1" {
              tunnel: w511 -> [_ w512]
              frame False {
              }
              frame True {
                n303 = stacked-sequence {
                  tunnel: w512 -> [_ _ _ _ _ _ _ w529]
                  frame #0 {
                    n304 = property on="Trap Delta (MHz)" class="DigNum (strict)"("Val(Sgnl)"="Offset 1 Start (MHz)") -> ()  [unwired: 2 in, 2 out]
                    n305 = Replace Array Subset(array=u32[] [0] ("Index Values"), new element="Offset 1 Set", index=0) -> (w513:u32[])
                    n306 = property on="Saved AOD Raster Scan Parameter Sets" class="Arr (strict)"("Index Values"=w513) -> ()  [unwired: 2 in, 2 out]
                  }
                  frame #1 {
                    n307 = Wait (ms)(milliseconds to wait=u32 200) -> ()  [unwired: 1 out]
                  }
                  frame #2 {
                    n308 = property on="Load parameters" class="Bool (strict)"("Val(Sgnl)"=TRUE ("Value (Signaling)")) -> ()  [unwired: 2 in, 2 out]
                  }
                  frame #3 {
                    n309 = Wait (ms)(milliseconds to wait=u32 200) -> ()  [unwired: 1 out]
                  }
                  frame #4 {
                    n310 = property on="Trap Raster Scan" class="Bool (strict)"("Val(Sgnl)"=TRUE ("Value (Signaling)")) -> ()  [unwired: 2 in, 2 out]
                  }
                  frame #5 {
                    n311 = Wait (ms)(milliseconds to wait=u32 2000) -> ()  [unwired: 1 out]
                  }
                  frame #6 {
                    n312 = while {
                      stop <- w526 stop-if-true
                      n313 = local read "Raster Scanning..."() -> (w528:bool)
                      n314 = local read "Saving..."() -> (w524:bool)
                      n315 = Wait (ms)(milliseconds to wait=u32 100) -> ()  [unwired: 1 out]
                      n316 = Not(x=w524) -> (.not. x?=w523:bool)
                      n317 = Not(x=w528) -> (.not. x?=w525:bool)
                      n318 = And(x=w525, y=w523) -> (x .and. y?=w526:bool)
                    }
                  }
                  frame #7 {
                    n319 = property on="Trap Delta (MHz)" class="DigNum (strict)"("Val(Sgnl)"=w529) -> ()  [unwired: 2 in, 2 out]
                  }
                }
              }
            }
          }
          frame #8 {
            n320 = local read "Save ave N"() -> (w531:dbl)
            n321 = case shown="False" "W/ Offset 2" {
              tunnel: w532 -> [_ w539]
              tunnel: w531 -> [_ w538]
              tunnel: w530 -> [w534 _]
              frame False {
                n322 = case shown="False" w534 {
                  frame False {
                    n323 = Multiply(x="Cal read wait (s)", y=u32 1000 ("milliseconds to wait")) -> (x*y=w536:u32)
                    n324 = Wait (ms)(milliseconds to wait=w536) -> ()  [unwired: 1 out]
                  }
                  frame True {
                  }
                }
              }
              frame True {
                n325 = stacked-sequence {
                  tunnel: w539 -> [_ _ _ _ _ _ _ _ _ w560 _ _]
                  tunnel: w538 -> [_ _ _ _ _ _ _ _ _ w558 _ _]
                  frame #0 {
                    n326 = property on="Save ave N" class="DigNum (strict)"("Val(Sgnl)"=1.0 ("Value (Signaling)")) -> ()  [unwired: 2 in, 2 out]
                  }
                  frame #1 {
                    n327 = Wait (ms)(milliseconds to wait=u32 500) -> ()  [unwired: 1 out]
                  }
                  frame #2 {
                    n328 = property on="Trap Delta (MHz)" class="DigNum (strict)"("Val(Sgnl)"="Offset 2 Start (MHz)") -> ()  [unwired: 2 in, 2 out]
                    n329 = Replace Array Subset(array=u32[] [0] ("Index Values"), new element="Offset 2 Set", index=0) -> (w544:u32[])
                    n330 = property on="Saved AOD Raster Scan Parameter Sets" class="Arr (strict)"("Index Values"=w544) -> ()  [unwired: 2 in, 2 out]
                  }
                  frame #3 {
                    n331 = Wait (ms)(milliseconds to wait=u32 500) -> ()  [unwired: 1 out]
                  }
                  frame #4 {
                    n332 = property on="Load parameters" class="Bool (strict)"("Val(Sgnl)"=TRUE ("Value (Signaling)")) -> ()  [unwired: 2 in, 2 out]
                  }
                  frame #5 {
                    n333 = Wait (ms)(milliseconds to wait=u32 500) -> ()  [unwired: 1 out]
                  }
                  frame #6 {
                    n334 = property on="Trap Raster Scan" class="Bool (strict)"("Val(Sgnl)"=TRUE ("Value (Signaling)")) -> ()  [unwired: 2 in, 2 out]
                  }
                  frame #7 {
                    n335 = Wait (ms)(milliseconds to wait=u32 2000) -> ()  [unwired: 1 out]
                  }
                  frame #8 {
                    n336 = while {
                      stop <- w553 stop-if-true
                      n337 = local read "Raster Scanning..."() -> (w556:bool)
                      n338 = local read "Saving..."() -> (w554:bool)
                      n339 = Wait (ms)(milliseconds to wait=u32 100) -> ()  [unwired: 1 out]
                      n340 = Not(x=w554) -> (.not. x?=w552:bool)
                      n341 = Not(x=w556) -> (.not. x?=w555:bool)
                      n342 = And(x=w555, y=w552) -> (x .and. y?=w553:bool)
                    }
                  }
                  frame #9 {
                    n343 = property on="Trap Delta (MHz)" class="DigNum (strict)"("Val(Sgnl)"=w560) -> ()  [unwired: 2 in, 2 out]
                    n344 = property on="Saved AOD Raster Scan Parameter Sets" class="Arr (strict)"("Index Values"=u32[] [0]) -> ()  [unwired: 2 in, 2 out]
                    n345 = property on="Save ave N" class="DigNum (strict)"("Val(Sgnl)"=w558) -> ()  [unwired: 2 in, 2 out]
                  }
                  frame #10 {
                    n346 = Wait (ms)(milliseconds to wait=u32 500) -> ()  [unwired: 1 out]
                  }
                  frame #11 {
                    n347 = property on="Load parameters" class="Bool (strict)"("Val(Sgnl)"=TRUE ("Value (Signaling)")) -> ()  [unwired: 2 in, 2 out]
                  }
                }
              }
            }
          }
          frame #9 {
            n348 = property on="Read Cal" class="Bool (strict)"("Val(Sgnl)"=TRUE ("Value (Signaling)")) -> ()  [unwired: 2 in, 2 out]
          }
          frame #10 {
            n349 = Wait (ms)(milliseconds to wait=u32 1000) -> ()  [unwired: 1 out]
          }
          frame #11 {
            n350 = property on="Fish for Tether" class="Bool (strict)"("Val(Sgnl)"=TRUE ("Value (Signaling)")) -> ()  [unwired: 2 in, 2 out]
          }
        }
        n351 = local write "Cal/Data Acq. Spot"(FALSE ("Cal/Data Acq. Spot")) -> ()
      }
      event "Dump Beads": Value Change {
        n352 = event-data() -> ()  [unwired: 1 in, 5 out]
        n353 = flat-sequence {
          tunnel: ["Dump spot flow on?"] -> w566
          tunnel: [w577] -> w567
          tunnel: w566 -> [w577]
          tunnel: w570 -> [w582]
          tunnel: w569 -> [w581]
          tunnel: [w579] -> w568
          tunnel: w567 -> [w579]
          tunnel: w568 -> [w592]
          frame #0 {
            w571 = FALSE ("Value (Signaling)")
            n354 = local read "Saving..."() -> (w573:bool)
            n355 = local write "Dump Beads"(FALSE ("Dump Beads")) -> ()
            n356 = property on="Inject Pump 3" class="Bool (strict)"("Val(Sgnl)"=w571) -> ()  [unwired: 2 in, 2 out]
            n357 = property on="Inject Pump 1" class="Bool (strict)"("Val(Sgnl)"=w571) -> ()  [unwired: 2 in, 2 out]
            n358 = local write "Stop Saving"(w573) -> ()
          }
          frame #1 {
            w574 = FALSE ("Fl. Triggered...")
            n359 = case shown="True" "Dump spot flow on?" {
